vi "SMS FlexRIO Example_FPGA_SMS.vi"() -> ()   [LabVIEW 2015]
uses:
  <vilib>/Platform/TimedLoop/XDataNode/timing_clust.ctl
  <vilib>/Platform/TimedLoop/XDataNode/nitl_modes.ctl
  <vilib>/Platform/TimedLoop/XDataNode/wakeup.ctl
  <vilib>/rvi/Emulation/niFpgaSctlEmulationGetInTimedLoop.vi
  <vilib>/rvi/Emulation/niFpgaEmulationReportErrorSimple.vi
  <vilib>/rvi/Emulation/niFpgaGetClockAttributes.vi
  <vilib>/rvi/Emulation/niFpgaCriticalErrorInLSC.vi
  <vilib>/rvi/eio/common/nirviEmuTemplateMethod_errors.vi
  <vilib>/rvi/Emulation/niFpgaProcessEmulError.vi
  <instrlib>/_niInstr/Basic Elements/v1/FPGA/Private/Count Up U64.vi
  <vilib>/rvi/DataTransferAndStorage/Container/Common/niFpgaContainerGetUniqueNameForEmu.vi
  <vilib>/rvi/DataTransferAndStorage/Container/Common/niFpgaContainerSetEmuInfo.vi
  <vilib>/rvi/eio/common/nirviEmuReportErrorAndStop.vi
  <vilib>/rvi/Emulation/niFpgaEmulationIsFPGAContextNoSignature.vi
  <vilib>/rvi/errors/niFpgaSetErrorForExecOnDevCompSimple.vi
  <vilib>/rvi/FIFO/Fifo_Resource/nirvififoEmulationSetSize.vi
  <vilib>/rvi/FIFO/Fifo_Resource/nirviFifoEmulationQueueMgr.vi
  <instcachedir>/0/nirviFifoEmulationQueueMgr_E5CAEC123FF24DC58D834DCA3CDAA9B5.lvgen/nirviFifoEmulationQueueMgr_E5CAEC123FF24DC58D834DCA3CDAA9B5_002.vi
  <vilib>/rvi/FIFO/Fifo_Resource/nirvififoEmulationDetermineInputValidOut.vi
  <vilib>/rvi/FIFO/Fifo_Resource/nirvififoEmulationCreateLock.vi
  <vilib>/rvi/FIFO/Fifo_Resource/nirvififoEmulationObtainLock.vi
  <vilib>/rvi/FIFO/Fifo_Resource/nirvififoEmulationReleaseLock.vi
  <vilib>/rvi/occurrence/nirviWaitOnOccurrenceBase.vi
  <vilib>/rvi/errors/nirviReportUnexpectedCaseInternalError.vi
  <vilib>/rvi/errors/nirviReportUnexpectedCaseInternalError (U32).vi
  <vilib>/rvi/interface/RandomDataEmulation/niFpgaRandomDataHandleErrors.vi
  <vilib>/Utility/error.llb/Clear Errors.vi
  <vilib>/Platform/TimedLoop/XDataNode/XDataNode.xnode
  <vilib>/eio/EIONode/EIONode.xnode
  <vilib>/rvi/LocalResourceManager/LocalResourceManager.xnode
  <vilib>/rvi/DataTransferAndStorage/Container/XNode/niFpgaContainer.xnode
  <vilib>/rvi/FIFO/Fifo_Resource/nirvififoEmulationWrite.vi
  <vilib>/rvi/interface/RandomDataEmulation/nirviRandomDataFpgaReadWriteTemplate.vi
  <vilib>/rvi/FIFO/Fifo_Resource/nirvififoEmulationRead.vi
  <vilib>/Platform/TimedLoop/XDataNode/XDNodeRunTimeDep.lvlib
  <instrlib>/_niInstr/Basic Elements/v1/FPGA/niInstr Basic Elements v1 FPGA.lvlib
panel:
  out "data valid":bool
  out "throughput reset":bool
  out "DMA Fault":bool
  in  "Capture Enabled":bool
  out "Throughput Count":u64
  in  "Throughput Reset Period":u64
  out "Capture Count":u64
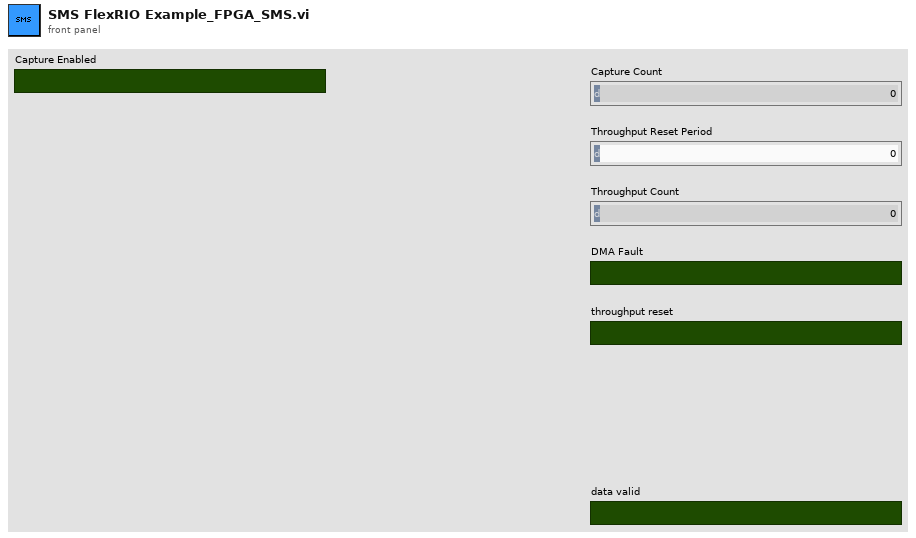
[diagram p1: front panel]
types:
  T1 = typedef "XDNodeRunTimeDep.lvlib/timing_clust.ctl" = cluster{"Expected End [f-1]":u64, "Actual End [f-1]":u64, "Finished Late? [f-1]":bool, "Expected End [i-1]":u64, "Actual End [i-1]":u64, "Finished Late? [i-1]":bool, "Expected Start [i]":u64, "Actual Start [i]":u64, "Expected Start [f]":u64, "Actual Start [f]":u64, "Source Name":string, "Structure Name":string, "Period":i64, "Deadline":i64, "Offset":i64, "Start":i64, "Priority":i32, "Timeout":i32, "Mode":T2, "Wakeup Reason":T3, "Error":errorcluster, "Source Type":string, "Secondary Source Type":string, "Global End Time":u64, "Global Start Time":u64, "Frame Duration":u64, "Iteration Duration":u64, "Assigned CPU":i32, "I/O Scan Engine Mode":u32}
  T2 = typedef "XDNodeRunTimeDep.lvlib/nitl_modes.ctl" = enum32{"No Change", "Process missed periods, maintain original phase", "Discard missed periods, maintain original phase", "Process missed periods, ignore original phase", "Discard missed periods, ignore original phase"}
  T3 = typedef "XDNodeRunTimeDep.lvlib/wakeup.ctl" = enum32{"Normal", "Aborted", "Asynchronous wakeup", "Timing source error", "Timed loop error", "Timeout"}
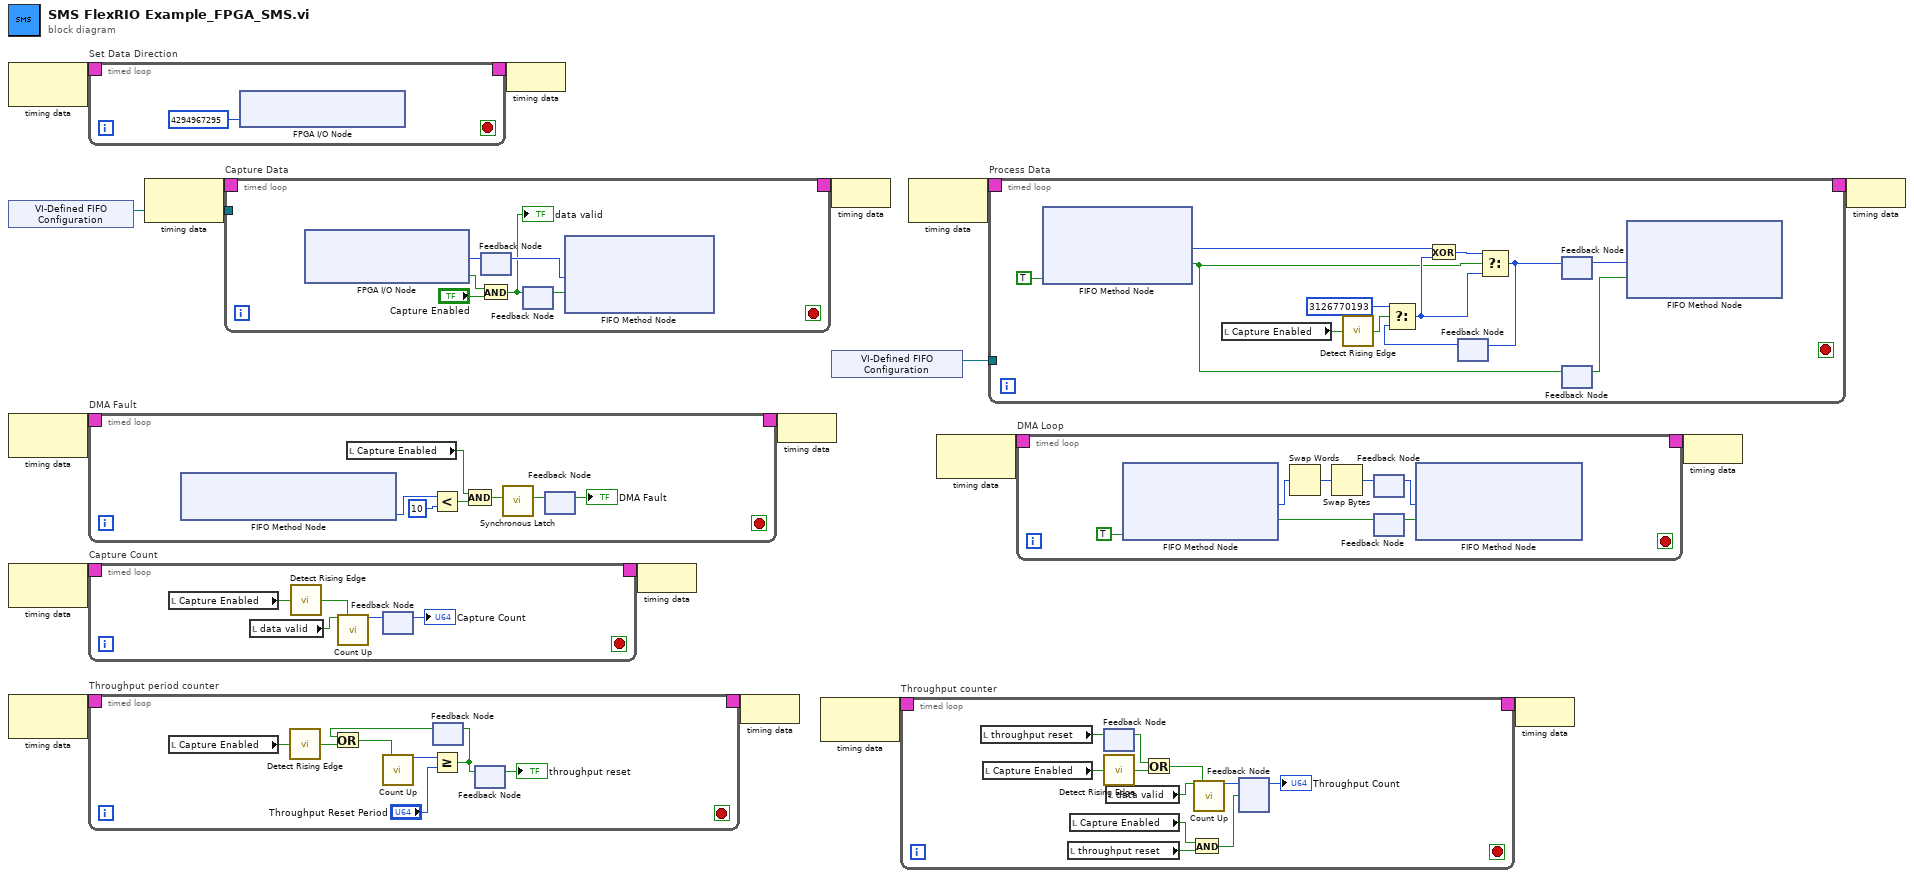
[diagram p0: block diagram]
diagram:
  n1 = node-c288() -> (w18:T1)  [unwired: 1 in]
  n2 = xnode "VI-Defined FIFO Configuration"() -> ("FIFO Out"=w12:refnum<k21>)
  n3 = node-c288() -> (w7:T1)  [unwired: 1 in]
  n4 = node-c288() -> (w9:T1)  [unwired: 1 in]
  n5 = node-c288() -> (w14:T1)  [unwired: 1 in]
  n6 = timed-loop "Set Data Direction" {
    timing: w18 -> [_]
    timing-out: [_] -> w17
    stop <- _ stop-if-true
    n7 = xnode "FPGA I/O Node"("IO Module\\SE_Data_Dir"=u32 4294967295 ("IO Module\\SE_Data_Dir")) -> ()  [unwired: 1 in, 1 out]
  }
  n8 = timed-loop "DMA Fault" {
    timing: w7 -> [_]
    timing-out: [_] -> w6
    stop <- _ stop-if-true
    n9 = xnode ("FIFO Method Node")() -> ("Number of Elements to Write"=w28:u32)  [unwired: 1 in, 1 out]
    n10 = local read "Capture Enabled"() -> (w25:bool)
    n11 = Less?(x=w28, y=u32 10) -> (x < y?=w23:bool)
    n12 = Compound Arithmetic op=AND(w25, w23) -> (w24:bool)
    n13 = call <instrlib>:"Synchronous Latch.vi"("set"=w24) -> ("out"=w26:bool)  [unwired: 10 in]
    n14 = feedback-in #1(w26) -> ()
    n15 = feedback #1() -> (→"DMA Fault":bool)  [unwired: 1 in]
  }
  n16 = timed-loop "Capture Count" {
    timing: w9 -> [_]
    timing-out: [_] -> w8
    stop <- _ stop-if-true
    n17 = local read "Capture Enabled"() -> (w34:bool)
    n18 = local read "data valid"() -> (w32:bool)
    n19 = call <instrlib>:"Detect Rising Edge.vi"("signal"=w34) -> ("edge detected"=w33:bool)  [unwired: 14 in]
    n20 = call-poly <instrlib>:"Count Up.vi"("increment"=w32, "reset"=w33) -> ("count out"=w35:u64)  [unwired: 13 in]
    n21 = feedback-in #2(w35) -> ()
    n22 = feedback #2() -> (→"Capture Count":u64)  [unwired: 1 in]
  }
  n23 = timed-loop "Throughput period counter" {
    timing: w14 -> [_]
    timing-out: [_] -> w13
    stop <- _ stop-if-true
    n24 = local read "Capture Enabled"() -> (w43:bool)
    n25 = call <instrlib>:"Detect Rising Edge.vi"("signal"=w43) -> ("edge detected"=w42:bool)  [unwired: 14 in]
    n26 = feedback #3() -> (w40:bool)  [unwired: 1 in]
    n27 = Or(x=w40, y=w42) -> (x .or. y?=w39:bool)
    n28 = call-poly <instrlib>:"Count Up.vi"("reset"=w39) -> ("count out"=w44:u64)  [unwired: 14 in]
    n29 = Greater Or Equal?(x=w44, y="Throughput Reset Period") -> (x >= y?=w41:bool)
    n30 = feedback-in #3(w41) -> ()
    n31 = feedback-in #4(w41) -> ()
    n32 = feedback #4() -> (→"throughput reset":bool)  [unwired: 1 in]
  }
  n33 = node-c288() -> (w16:T1)  [unwired: 1 in]
  n34 = timed-loop "Capture Data" {
    timing: w16 -> [_]
    timing-out: [_] -> w15
    tunnel: w12 -> [_]
    stop <- _ stop-if-true
    n35 = xnode "FPGA I/O Node"() -> ("IO Module\\SE_Data_Rd"=w53:u32, "IO Module\\SE_PFI1_Rd"=w51:bool)  [unwired: 2 in, 2 out]
    n36 = feedback-in #5(w53) -> ()
    n37 = feedback #5() -> (w52:u32)  [unwired: 1 in]
    n38 = And(x=w51, y="Capture Enabled") -> (x .and. y?=w49:bool)
    "data valid" <- w49
    n39 = feedback-in #6(w49) -> ()
    n40 = feedback #6() -> (w50:bool)  [unwired: 1 in]
    n41 = xnode ("FIFO Method Node")("Element"=w52, "Input Valid"=w50) -> ()  [unwired: 1 in, 2 out]
  }
  n42 = node-c288(w17) -> ()
  n43 = node-c288(w8) -> ()
  n44 = node-c288(w13) -> ()
  n45 = node-c288(w6) -> ()
  n46 = node-c288() -> (w11:T1)  [unwired: 1 in]
  n47 = node-c288(w15) -> ()
  n48 = xnode "VI-Defined FIFO Configuration"() -> ("FIFO Out"=w3:refnum<k21>)
  n49 = timed-loop "Throughput counter" {
    timing: w11 -> [_]
    timing-out: [_] -> w10
    stop <- _ stop-if-true
    n50 = local read "throughput reset"() -> (w62:bool)
    n51 = local read "Capture Enabled"() -> (w61:bool)
    n52 = local read "throughput reset"() -> (w58:bool)
    n53 = local read "Capture Enabled"() -> (w60:bool)
    n54 = feedback-in #7(w62) -> ()
    n55 = feedback #7() -> (w57:bool)  [unwired: 1 in]
    n56 = call <instrlib>:"Detect Rising Edge.vi"("signal"=w61) -> ("edge detected"=w59:bool)  [unwired: 14 in]
    n57 = local read "data valid"() -> (w56:bool)
    n58 = Or(x=w57, y=w59) -> (x .or. y?=w65:bool)
    n59 = And(x=w60, y=w58) -> (x .and. y?=w66:bool)
    n60 = call-poly <instrlib>:"Count Up.vi"("increment"=w56, "reset"=w65) -> ("count out"=w64:u64)  [unwired: 13 in]
    n61 = feedback #8() -> (→"Throughput Count":u64)  [unwired: 1 in]
    n62 = feedback-in #8(w64, w66) -> ()
  }
  n63 = node-c288() -> (w5:T1)  [unwired: 1 in]
  n64 = node-c288() -> (w2:T1)  [unwired: 1 in]
  n65 = timed-loop "Process Data" {
    timing: w5 -> [_]
    timing-out: [_] -> w4
    tunnel: w3 -> [_]
    stop <- _ stop-if-true
    n66 = xnode ("FIFO Method Node")("Ready for Output"=TRUE) -> ("Element"=w77:u32, "Output Valid"=w72:bool)  [unwired: 1 in, 1 out]
    n67 = local read "Capture Enabled"() -> (w70:bool)
    n68 = call <instrlib>:"Detect Rising Edge.vi"("signal"=w70) -> ("edge detected"=w69:bool)  [unwired: 14 in]
    n69 = feedback #9() -> (w79:u32)  [unwired: 1 in]
    n70 = Select(t=u32 3126770193, s=w69, f=w79) -> (s? t:f=w74:u32)
    n71 = Exclusive Or(1:w74, 2:w77) -> (0:w76:u32)
    n72 = Select(t=w76, s=w72, f=w74) -> (s? t:f=w75:u32)
    n73 = feedback-in #9(w75) -> ()
    n74 = feedback #10() -> (w73:u32)  [unwired: 1 in]
    n75 = feedback-in #10(w75) -> ()
    n76 = feedback-in #11(w72) -> ()
    n77 = feedback #11() -> (w71:bool)  [unwired: 1 in]
    n78 = xnode ("FIFO Method Node")("Element"=w73, "Input Valid"=w71) -> ()  [unwired: 1 in, 2 out]
  }
  n79 = timed-loop "DMA Loop" {
    timing: w2 -> [_]
    timing-out: [_] -> w1
    stop <- _ stop-if-true
    n80 = xnode ("FIFO Method Node")("Ready for Output"=TRUE) -> ("Element"=w89:u32, "Output Valid"=w88:bool)  [unwired: 1 in, 1 out]
    n81 = Swap Words(1:w89) -> (0:w86:u32)
    n82 = Swap Bytes(anything=w86) -> (byte swapped=w85:u32)
    n83 = feedback-in #12(w85) -> ()
    n84 = feedback #12() -> (w84:u32)  [unwired: 1 in]
    n85 = feedback-in #13(w88) -> ()
    n86 = feedback #13() -> (w83:bool)  [unwired: 1 in]
    n87 = xnode ("FIFO Method Node")("Element"=w84, "Input Valid"=w83) -> ()  [unwired: 1 in, 2 out]
  }
  n88 = node-c288(w10) -> ()
  n89 = node-c288(w1) -> ()
  n90 = node-c288(w4) -> ()
